vi "Bit Inverter.vi"(11 "Bit stream in":u8[](array[numeric])=[0, 0, 0, 0, 0, 0, 0, 0, 0, 0]) -> (3 "Inverted bit stream out":u8[](array[numeric]))   [LabVIEW 2019]
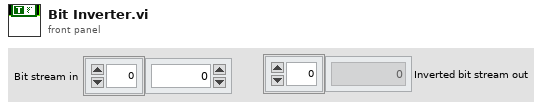
[diagram p1: front panel]
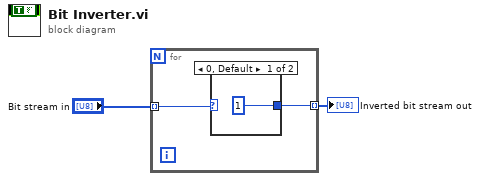
[diagram p0: block diagram]
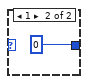
[diagram p2: hidden frame]
diagram:
  n1 = for {
    tunnel: "Bit stream in" -> [w4] mode=indexing
    tunnel: [w3] -> w1 mode=indexing
    n2 = case shown="0, Default" w4 {
      tunnel: [u8 1 ("Numeric") u8 0 ("Numeric")] -> w3
      frame 0, Default {
      }
      frame 1 {
      }
    }
  }
  "Inverted bit stream out" <- w1
